vi "robot - Draw Joint.vi"(6 "Light Direction":dbl(knob)=314.8880943229338 scale=0.0..360.0 scale format="%.1f", 7 "Enhance Style":bool, 9 "Color":u32(colorbox)=13395558, 10 "Rectangle":T1, 11 "Picture In":picture) -> (3 "Picture Out":picture)   [LabVIEW 2023]
doc: "This VI draws a single joint either flat, or highlighted for depth."
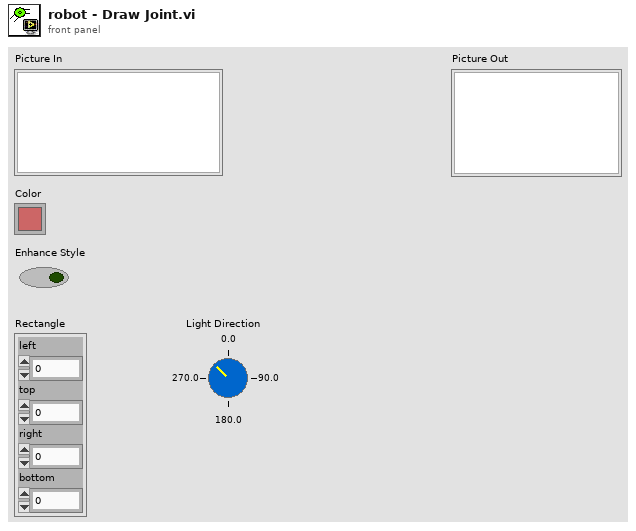
[diagram p1: front panel]
types:
  T1 = cluster{"left":i16, "top":i16, "right":i16, "bottom":i16}
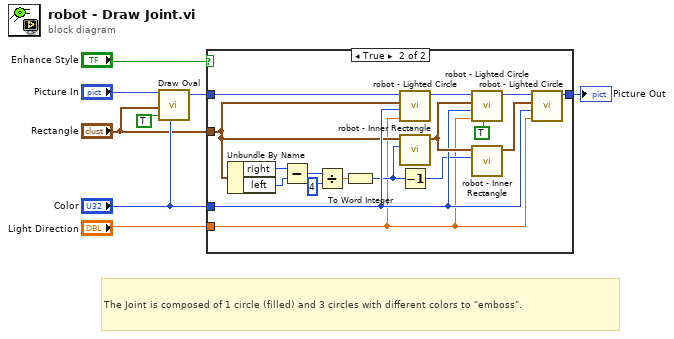
[diagram p0: block diagram]
diagram:
  # "The Joint is composed of 1 circle (filled) and 3 circles with different colors to \"emboss\"."
  n1 = call <vilib>:"Draw Oval.vi"("picture"="Picture In", "rect"="Rectangle", "fill?(F)"=TRUE, "color(black)"="Color") -> ("new picture"=w5:picture)  [unwired: 5 in]
  n2 = case shown="True" "Enhance Style" {
    tunnel: w5 -> [w9 w26]
    tunnel: [w9 w22] -> w1
    tunnel: "Color" -> [_ w21]
    tunnel: "Rectangle" -> [_ w11]
    tunnel: "Light Direction" -> [_ w10]
    frame False {
    }
    frame True {
      n3 = Unbundle By Name(w11) -> ("right"=w18:i16, "left"=w17:i16)
      n4 = Subtract(x=w18, y=w17) -> (x-y=w15:i16)
      n5 = Divide(x=w15, y=4) -> (x/y=w14:dbl)
      n6 = To Word Integer(number=w14) -> (16bit integer=w13:i16)
      n7 = call "robot - Lighted Circle.vi"("Light Direction"=w10, "Color"=w21, "Pict Rect"=w11, "Picture In"=w26) -> ("Picture Out"=w25:picture)  [unwired: 7 in]
      n8 = call "robot - Inner Rectangle.vi"("size/2"=w13, "Rectangle In"=w11) -> ("Rectangle Out"=w24:T1)  [unwired: 9 in]
      n9 = Decrement(x=w13) -> (x-1=w12:i16)
      n10 = call "robot - Lighted Circle.vi"("Lowered"=TRUE, "Light Direction"=w10, "Color"=w21, "Pict Rect"=w24, "Picture In"=w25) -> ("Picture Out"=w23:picture)  [unwired: 6 in]
      n11 = call "robot - Inner Rectangle.vi"("size/2"=w12, "Rectangle In"=w24) -> ("Rectangle Out"=w20:T1)  [unwired: 9 in]
      n12 = call "robot - Lighted Circle.vi"("Light Direction"=w10, "Color"=w21, "Pict Rect"=w20, "Picture In"=w23) -> ("Picture Out"=w22:picture)  [unwired: 7 in]
    }
  }
  "Picture Out" <- w1
